vi "SyntaxCheckToken.vi"(6 "error in":errorcluster, 7 "Error Index In":i32, 8 "Funcion":string, 9 "SyntaxChek In":string[](array[string])) -> (0 "error out":errorcluster, 1 "Error Index Out":i32, 3 "SyntaxChek Out":string[](array[string]))   [LabVIEW 2014, in "MathLoop.lvlib"]
uses:
  MathLoop.lvlib
  <vilib>/regexp/Match Regular Expression.xnode
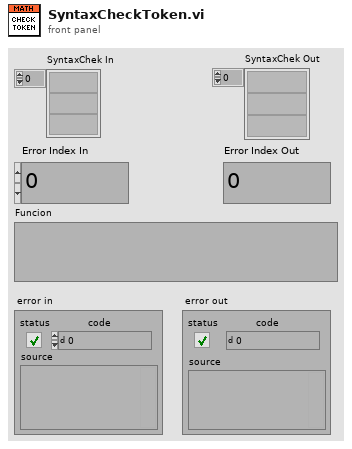
[diagram p1: front panel]
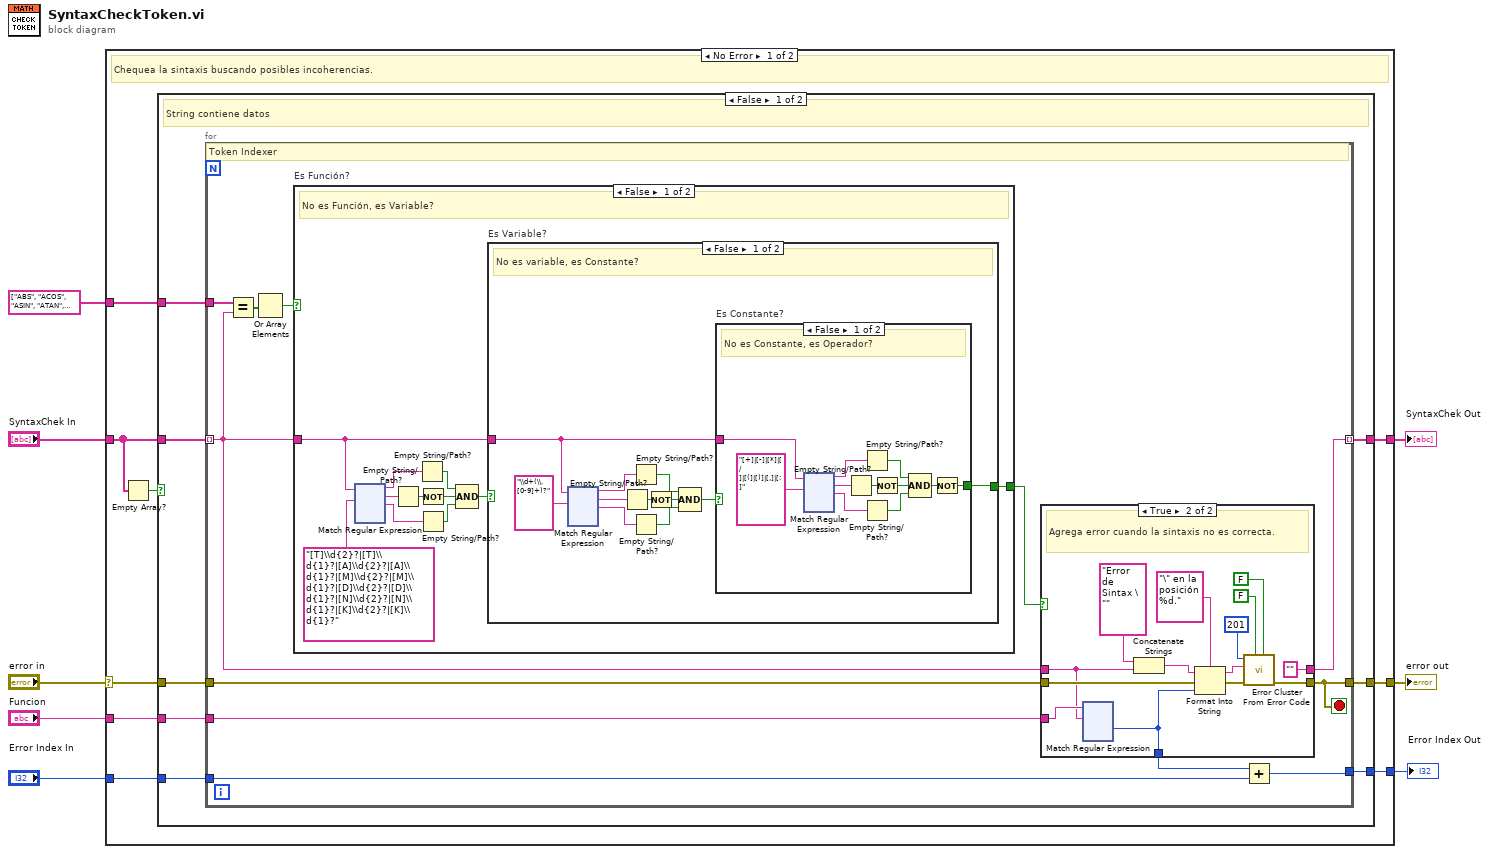
[diagram p0: block diagram]
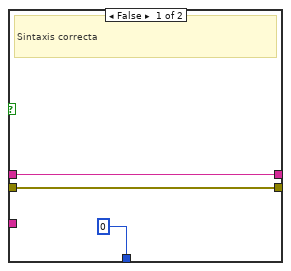
[diagram p2: hidden frame]
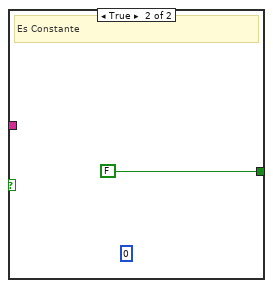
[diagram p3: hidden frame]
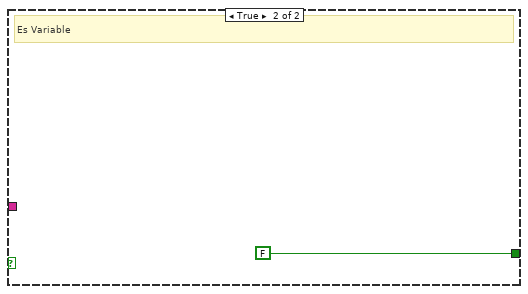
[diagram p4: hidden frame]
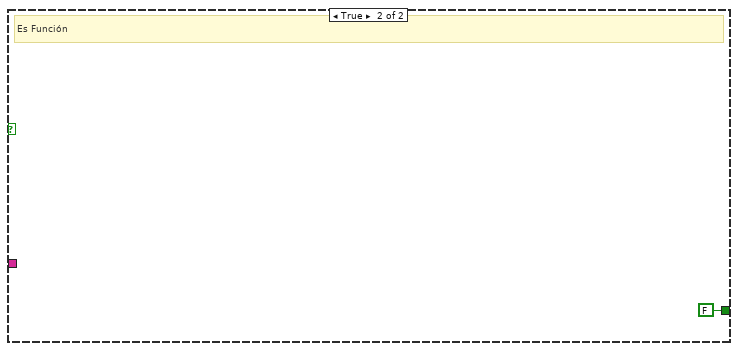
[diagram p5: hidden frame]
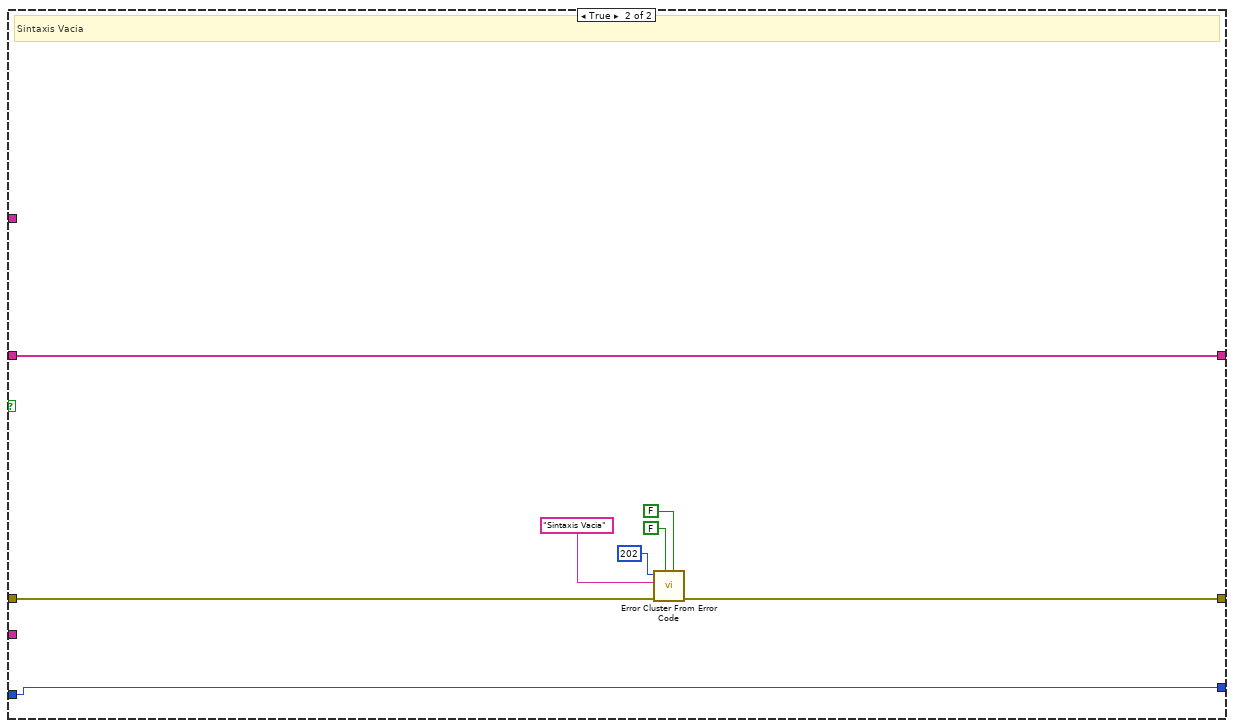
[diagram p6: hidden frame]
diagram:
  n1 = case shown="No Error" "error in" {
    selector: "error in" -> [w17 w557]
    tunnel: [w16 w557] -> w7
    tunnel: "SyntaxChek In" -> [w14 w556]
    tunnel: string[] ["ABS", "ACOS", "ASIN", "ATAN", "CEIL", "COS", "EXP", "FLOOR", "GETA", "GETM", "GRAD2RAD", "LOG", "MAX", "MIN", "NEG", "POW", "RAD2GRAD", "ROUND", "SIN", "SQRT", "TAN", "TRUNC"] ("Funciones") -> [w13 _]
    tunnel: [w12 w556] -> w4
    tunnel: "Error Index In" -> [w11 w555]
    tunnel: [w10 w555] -> w2
    tunnel: "Funcion" -> [w9 _]
    frame No Error {
      # "Chequea la sintaxis buscando posibles incoherencias."
      n2 = Empty Array?(array=w14) -> (empty?=w15:bool)
      n3 = case shown="False" w15 {
        tunnel: w14 -> [w25 w548]
        tunnel: w13 -> [w24 _]
        tunnel: w17 -> [w23 w549]
        tunnel: [w22 w550] -> w16
        tunnel: [w21 w548] -> w12
        tunnel: w11 -> [w20 w547]
        tunnel: [w19 w547] -> w10
        tunnel: w9 -> [w18 _]
        frame False {
          # "String contiene datos"
          n4 = for {
            tunnel: w25 -> [w30] mode=indexing
            tunnel: w24 -> [w32]
            tunnel: w23 -> [w35]
            tunnel: [w34] -> w22
            tunnel: [w31] -> w21 mode=indexing
            tunnel: w20 -> [w29]
            tunnel: [w28] -> w19
            tunnel: w18 -> [w27]
            stop <- w34 stop-if-true
            # "Token Indexer"
            n5 = Equal?(x=w32, y=w30) -> (x = y?=w37:bool[])
            n6 = Or Array Elements(Boolean array=w37) -> (logical OR=w36:bool)
            n7 = case "Es Función?" shown="False" w36 {
              tunnel: w30 -> [w169 _]
              tunnel: [w171 FALSE] -> w33
              frame False {
                # "No es Función, es Variable?"
                n8 = xnode "Match Regular Expression"("input string"=w169, "regular expression"="[T]\\d{2}?|[T]\\d{1}?|[A]\\d{2}?|[A]\\d{1}?|[M]\\d{2}?|[M]\\d{1}?|[D]\\d{2}?|[D]\\d{1}?|[N]\\d{2}?|[N]\\d{1}?|[K]\\d{2}?|[K]\\d{1}?") -> ("before match"=w178:string, "whole match"=w175:string, "after match"=w176:string)  [unwired: 4 in, 2 out]
                n9 = Empty String/Path?(string/path=w175) -> (empty?=w177:bool)
                n10 = Empty String/Path?(string/path=w178) -> (empty?=w174:bool)
                n11 = Not(x=w177) -> (.not. x?=w173:bool)
                n12 = Empty String/Path?(string/path=w176) -> (empty?=w172:bool)
                n13 = Compound Arithmetic op=AND(w174, w173, w172) -> (w170:bool)
                n14 = case "Es Variable?" shown="False" w170 {
                  tunnel: w169 -> [w181 _]
                  tunnel: [w182 FALSE] -> w171
                  frame False {
                    # "No es variable, es Constante?"
                    n15 = xnode "Match Regular Expression"("input string"=w181, "regular expression"="\\d+(\\.[0-9]+)?") -> ("before match"=w189:string, "whole match"=w186:string, "after match"=w187:string)  [unwired: 4 in, 2 out]
                    n16 = Empty String/Path?(string/path=w186) -> (empty?=w188:bool)
                    n17 = Empty String/Path?(string/path=w189) -> (empty?=w185:bool)
                    n18 = Empty String/Path?(string/path=w187) -> (empty?=w183:bool)
                    n19 = Not(x=w188) -> (.not. x?=w184:bool)
                    n20 = Compound Arithmetic op=AND(w185, w184, w183) -> (w180:bool)
                    n21 = case "Es Constante?" shown="False" w180 {
                      tunnel: w181 -> [w193 _]
                      tunnel: [w192 FALSE] -> w182
                      frame False {
                        # "No es Constante, es Operador?"
                        n22 = xnode "Match Regular Expression"("input string"=w193, "regular expression"="[+]|[-]|[*]|[/]|[(]|[)]|[,]|[:]") -> ("before match"=w200:string, "whole match"=w197:string, "after match"=w198:string)  [unwired: 4 in, 2 out]
                        n23 = Empty String/Path?(string/path=w197) -> (empty?=w199:bool)
                        n24 = Empty String/Path?(string/path=w200) -> (empty?=w196:bool)
                        n25 = Empty String/Path?(string/path=w198) -> (empty?=w194:bool)
                        n26 = Not(x=w199) -> (.not. x?=w195:bool)
                        n27 = Compound Arithmetic op=AND(w196, w195, w194) -> (w191:bool)
                        n28 = Not(x=w191) -> (.not. x?=w192:bool)
                      }
                      frame True {
                        (unwired) 0 ("offset past match")
                        # "Es Constante"
                      }
                    }
                  }
                  frame True {
                    # "Es Variable"
                  }
                }
              }
              frame True {
                # "Es Función"
              }
            }
            n29 = case shown="True" w33 {
              tunnel: w35 -> [w40 w45]
              tunnel: [w40 w44] -> w34
              tunnel: w30 -> [w39 w42]
              tunnel: [w39 "" ("String")] -> w31
              tunnel: w27 -> [_ w43]
              tunnel: [0 w41] -> w26
              frame False {
                # "Sintaxis correcta"
              }
              frame True {
                # "Agrega error cuando la sintaxis no es correcta."
                n30 = xnode "Match Regular Expression"("input string"=w43, "regular expression"=w42) -> ("offset past match"=w41:i32)  [unwired: 4 in, 4 out]
                n31 = Concatenate Strings("Error de Sintax \"" ("error message (\"\")"), w42) -> (w47:string)
                n32 = Format Into String(format string="\" en la posición %d.", initial string=w47, error in=w45, w41) -> (resulting string=w48:string, error out=w49:errorcluster)
                n33 = call <vilib>:"Error Cluster From Error Code.vi"("is warning? (False)"=FALSE, "show call chain? (False)"=FALSE, "error in (no error)"=w49, "error message (\"\")"=w48, "error code (0)"=201) -> ("error out"=w44:errorcluster)  [unwired: 4 in]
              }
            }
            n34 = Add(x=w26, y=w29) -> (x+y=w28:i32)
          }
        }
        frame True {
          # "Sintaxis Vacia"
          n35 = call <vilib>:"Error Cluster From Error Code.vi"("is warning? (False)"=FALSE, "show call chain? (False)"=FALSE, "error in (no error)"=w549, "error message (\"\")"="Sintaxis Vacia" ("error message (\"\")"), "error code (0)"=202) -> ("error out"=w550:errorcluster)  [unwired: 4 in]
        }
      }
    }
    frame Error {
    }
  }
  "error out" <- w7
  "SyntaxChek Out" <- w4
  "Error Index Out" <- w2
